vi "apply key value pairs.vi"(8 "error in":errorcluster, 9 "values":string[](array[string]), 10 "keys":string[](array[string]), 11 "fixed channel tag bus module in":refnum<class "fixed channel tag bus module.lvclass">) -> (0 "error out":errorcluster, 3 "fixed channel tag bus module out":refnum<class "fixed channel tag bus module.lvclass">)   [LabVIEW 2013, in "fixed channel tag bus module.lvclass"]
uses:
  fixed channel tag bus module.lvclass
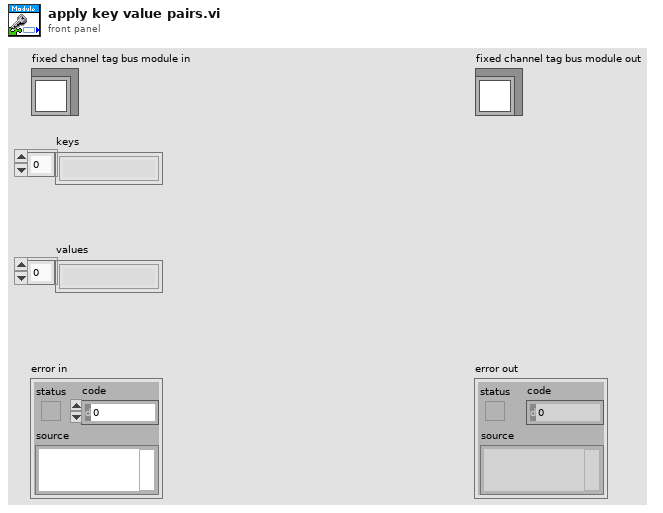
[diagram p1: front panel]
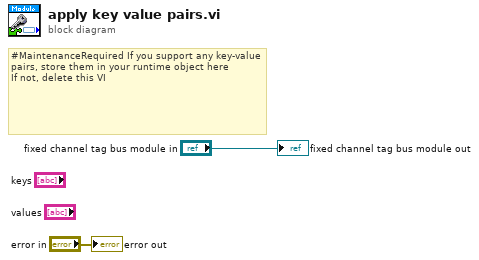
[diagram p0: block diagram]
diagram:
  # "#MaintenanceRequired If you support any key-value pairs, store them in your runtime object here\nIf not, delete this VI"
  "error out" <- "error in"
  "fixed channel tag bus module out" <- "fixed channel tag bus module in"
